vi "set_instruments (SubVI).vi"(0 "Process list":T5, 1 "Flash lamp settings:":T4={"Output channel (for flashing)"="Dev4/ao0", "Loop iteration"=0, "Path"=path "", "Flash lamp\n settings:"={"Flash lamp?"=FALSE, "Number of cyles\nbetween flashes"=3, "# Pulses"=35, "Stop flashing \nbelow thresh?"=FALSE, "Stop threshold"=0.001, "Pulse voltage?"=FALSE, "Pulse length (ms)"=0.001, "Pulse amp (V)"=0.001}}, 2 "signal type":T1(ring), 4 "electrodes reference":refnum<vi>, 5 "instrument config":T3, 6 "Num samples":i32, 7 "small amp":dbl=1.0 format="%0.2p", 9 "Volt vs pos array":cluster{dbl, dbl}[](array[cluster]), 10 "wfm?":bool, 11 "small amp freq":dbl=10.0 format="%0.2p", 12 "User Def. Wfm Name":string="RANDFREQ", 13 "Add small amp?":bool) -> (14 "Curr threshold":dbl, 18 "DC volts arr":dbl[](array[numeric]), 19 "instrum out":T2)   [LabVIEW 2016]
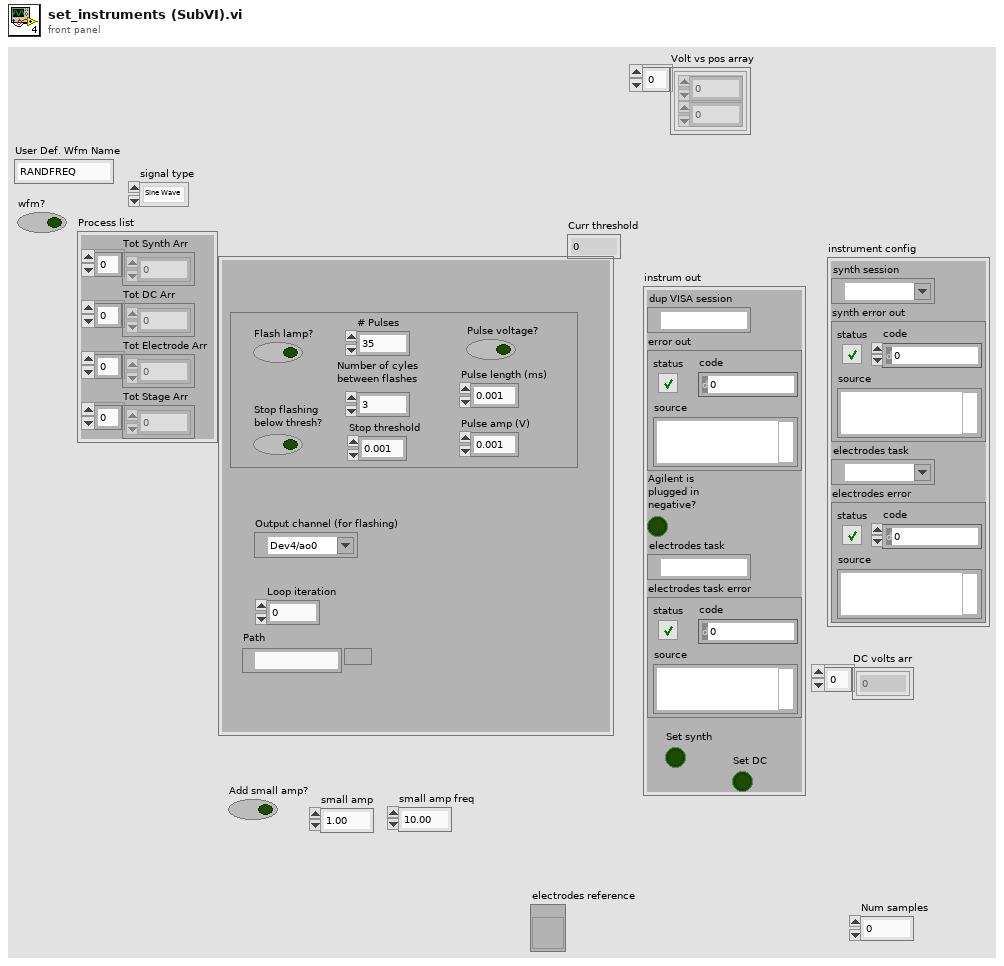
[diagram p1: front panel]
types:
  T1 = enum16{"Sine Wave", "Triangle Wave", "Square Wave", "Sawtooth Wave"}
  T2 = cluster{"dup VISA session":refnum<visa-resource-name>, "error out":errorcluster, "Agilent is \nplugged in \nnegative?":bool, "electrodes task":refnum<k21>, "electrodes task error":errorcluster, "Set synth":bool, "Set DC":bool}
  T3 = cluster{"synth session":refnum<visa-resource-name>, "synth error out":errorcluster, "electrodes task":refnum<k21>, "electrodes error":errorcluster}
  T4 = cluster{"Output channel (for flashing)":tag, "Loop iteration":i32, "Path":path, "Flash lamp\n settings:":cluster{"Flash lamp?":bool, "Number of cyles\nbetween flashes":i32, "# Pulses":i32, "Stop flashing \nbelow thresh?":bool, "Stop threshold":dbl, "Pulse voltage?":bool, "Pulse length (ms)":dbl, "Pulse amp (V)":dbl}}
  T5 = cluster{"Tot Synth Arr":dbl[], "Tot DC Arr":dbl[], "Tot Electrode Arr":dbl[], "Tot Stage Arr":dbl[]}
  T6 = cluster{"Flash lamp?":bool, "Number of cyles\nbetween flashes":i32, "# Pulses":i32, "Stop flashing \nbelow thresh?":bool, "Stop threshold":dbl, "Pulse voltage?":bool, "Pulse length (ms)":dbl, "Pulse amp (V)":dbl}
  T7 = cluster{"VISA resource name out":refnum<visa-resource-name>, "error out":errorcluster, "Agilent is \nplugged in \nnegative?":bool, "electrodes task":refnum<k21>, "electrodes error":errorcluster, "wfm?":bool, "Agilent is \nplugged in \nnegative?":bool}
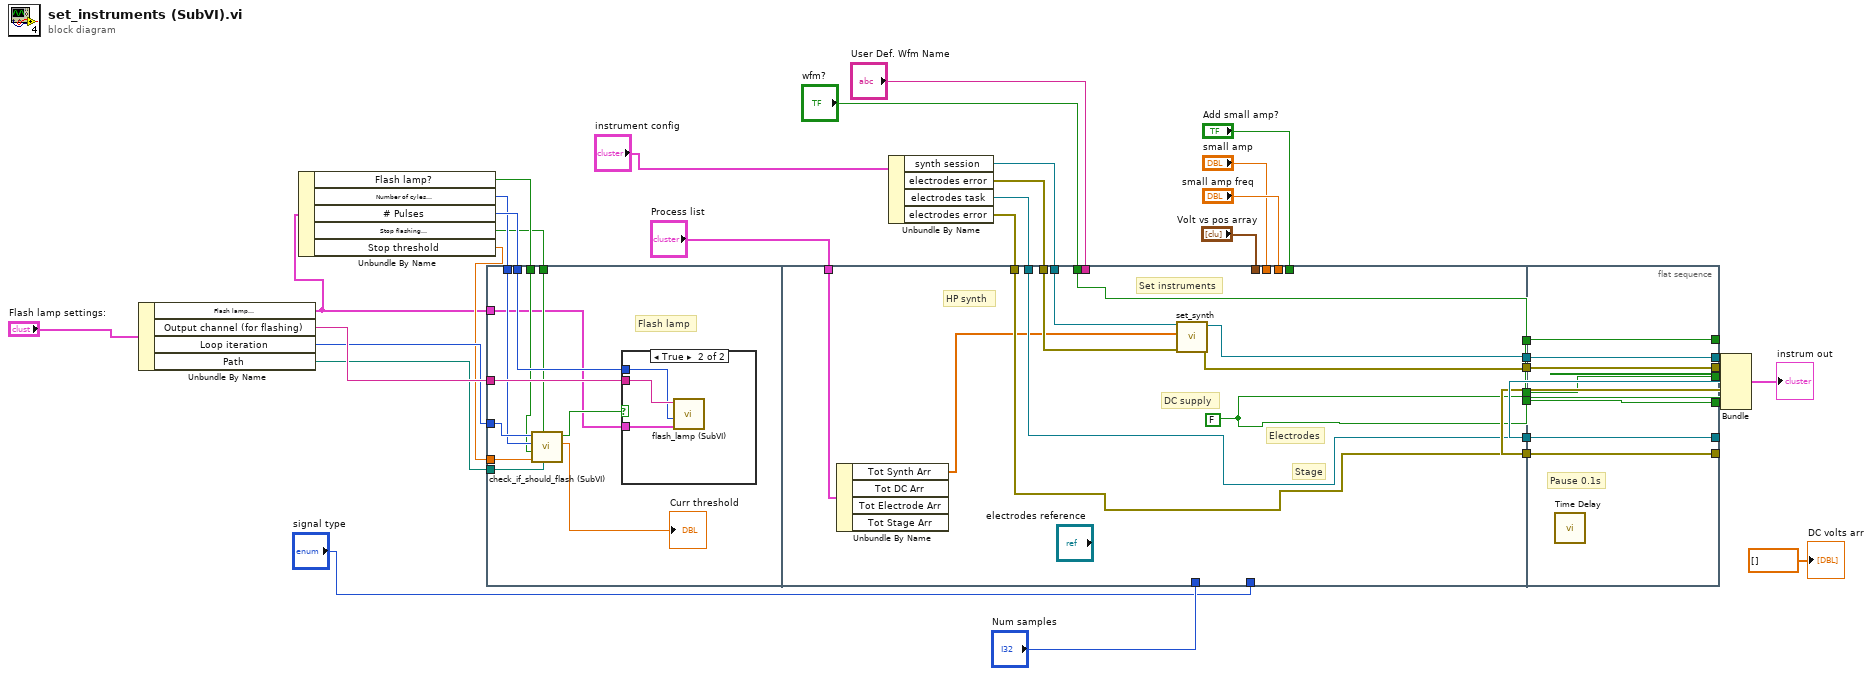
[diagram p0: block diagram]
diagram:
  n1 = Unbundle By Name("Flash lamp settings:") -> ("Flash lamp\n settings:"=w3:T6, "Output channel (for flashing)"=w38:tag, "Loop iteration"=w36:i32, "Path"=w33:path)
  n2 = Unbundle By Name(w3) -> ("Flash lamp?"=w34:bool, "Number of cyles\nbetween flashes"=w35:i32, "# Pulses"=w37:i32, "Stop flashing \nbelow thresh?"=w31:bool, "Stop threshold"=w32:dbl)
  n3 = flat-sequence {
    tunnel: w38 -> [w51]
    tunnel: w37 -> [w50]
    tunnel: w36 -> [w49]
    tunnel: w35 -> [w48]
    tunnel: w34 -> [w47]
    tunnel: w33 -> [w46]
    tunnel: w32 -> [w45]
    tunnel: w31 -> [w44]
    tunnel: w3 -> [w41]
    tunnel: "Process list" -> [w64]
    tunnel: w30 -> [w59]
    tunnel: w29 -> [w58]
    tunnel: w26 -> [w61]
    tunnel: w27 -> [w60]
    tunnel: [w61] -> w19
    tunnel: [w56] -> w18
    tunnel: [w57] -> w17
    tunnel: [w62] -> w16
    tunnel: [w60] -> w15
    tunnel: [w62] -> w14
    tunnel: [w63] -> w12
    tunnel: "Num samples" -> [_]
    tunnel: "wfm?" -> [w63]
    tunnel: "User Def. Wfm Name" -> [_]
    tunnel: "small amp freq" -> [_]
    tunnel: "small amp" -> [_]
    tunnel: "Add small amp?" -> [_]
    tunnel: "Volt vs pos array" -> [_]
    tunnel: "signal type" -> [_]
    tunnel: [w67] -> w21
    tunnel: [w68] -> w23
    tunnel: [w69] -> w24
    tunnel: [w70] -> w25
    tunnel: [w71] -> w22
    tunnel: w19 -> [w71]
    tunnel: w18 -> [w70]
    tunnel: w17 -> [w69]
    tunnel: w16 -> [w68]
    tunnel: w15 -> [w67]
    tunnel: w14 -> [w66]
    tunnel: [w66] -> w13
    tunnel: [w65] -> w11
    tunnel: w12 -> [w65]
    frame #0 {
      # "Flash lamp"
      n4 = call "check_if_should_flash (SubVI).vi"("Path"=w46, "Stop below threshold"=w44, "Stop threshold"=w45, "Flash lamp?"=w47, "Number of cyles\nbetween flashes"=w48, "Loop iteration"=w49) -> ("Curr threshold"=→"Curr threshold":dbl, "Should flash"=w43:bool)  [unwired: 4 in]
      n5 = case shown="True" w43 {
        tunnel: w51 -> [_ w54]
        tunnel: w50 -> [_ w53]
        tunnel: w41 -> [_ w52]
        frame False {
        }
        frame True {
          n6 = call "flash_lamp (SubVI).vi"("Flash lamp\n settings:"=w52, "# Pulses in"=w53, "Output channel (for flashing)"=w54) -> ()  [unwired: 9 in]
        }
      }
    }
    frame #1 {
      w62 = FALSE ("Agilent is \nplugged in \nnegative?")
      # "Stage"
      # "Electrodes"
      # "DC supply"
      # "HP synth"
      # "Set instruments"
      n7 = Unbundle By Name(w64) -> ("Tot Synth Arr"=w55:dbl[])  [unwired: 3 out]
      n8 = call "set_synth.vi"("error in (no error)"=w58, "Tot Synth Arr"=w55, "VISA resource name"=w59) -> ("error out"=w57:errorcluster, "VISA resource name out"=w56:refnum<visa-resource-name>)  [unwired: 7 in]
    }
    frame #2 {
      # "Pause 0.1s"
      n9 = call "Time Delay"() -> ()  [unwired: 11 in, 1 out]
    }
  }
  n10 = Unbundle By Name("instrument config") -> ("synth session"=w30:refnum<visa-resource-name>, "electrodes error"=w29:errorcluster, "electrodes task"=w26:refnum<k21>, "electrodes error"=w27:errorcluster)
  n11 = Bundle("VISA resource name out"=w25, "error out"=w24, "Agilent is \nplugged in \nnegative?"=w23, "electrodes task"=w22, "electrodes error"=w21, "wfm?"=w11, "Agilent is \nplugged in \nnegative?"=w13) -> (→"instrum out":T7)  [unwired: 1 in]
  "DC volts arr" <- dbl[] [] ("DC volts arr")
